vi "AWG_init.vi"(1 "Initialize?":u64, 2 "Inst_param":T1) -> (0 "error out":errorcluster)   [LabVIEW 2013]
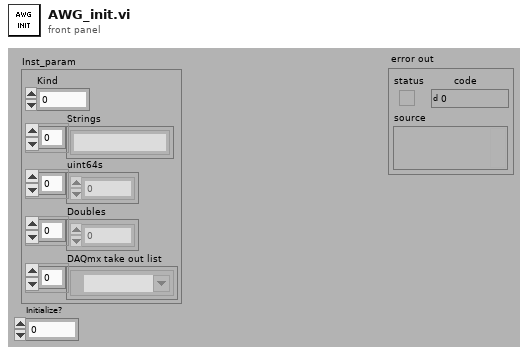
[diagram p1: front panel]
types:
  T1 = cluster{"Kind":u16, "Strings":string[], "uint64s":u64[], "Doubles":dbl[], "DAQmx take out list":refnum<k21>[]}
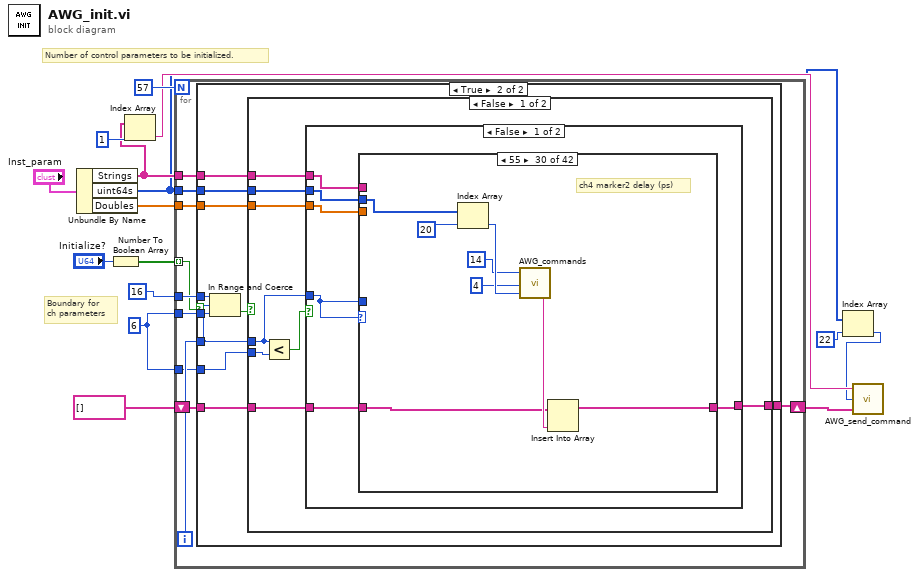
[diagram p0: block diagram]
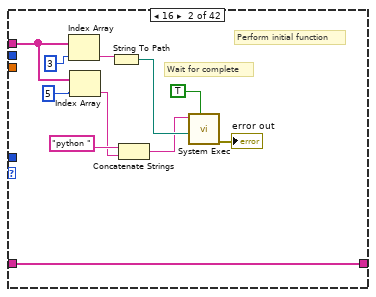
[diagram p4: hidden frame]
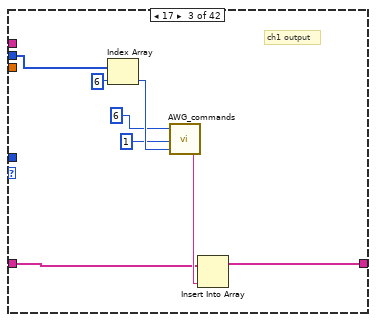
[diagram p5: hidden frame]
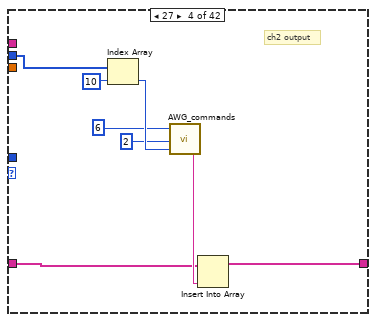
[diagram p6: hidden frame]
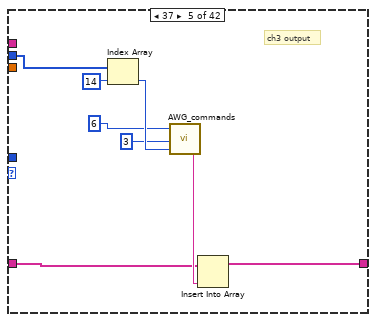
[diagram p7: hidden frame]
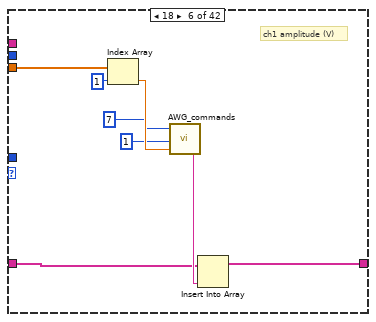
[diagram p8: hidden frame]
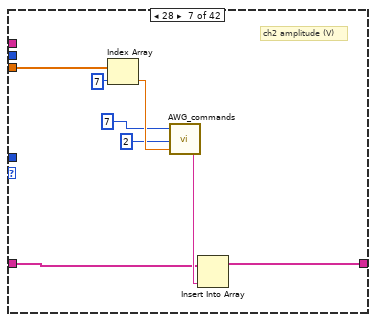
[diagram p9: hidden frame]
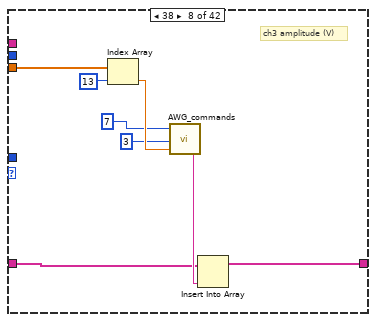
[diagram p10: hidden frame]
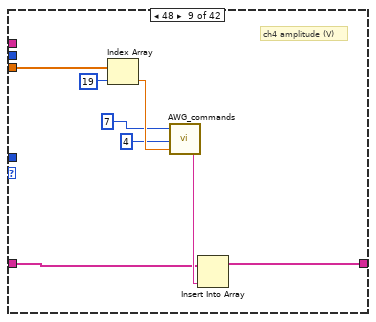
[diagram p11: hidden frame]
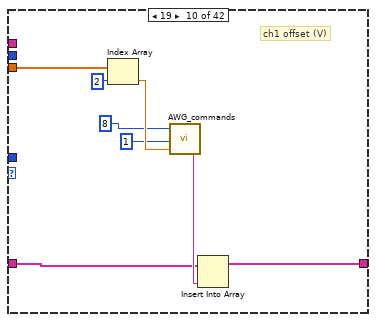
[diagram p12: hidden frame]
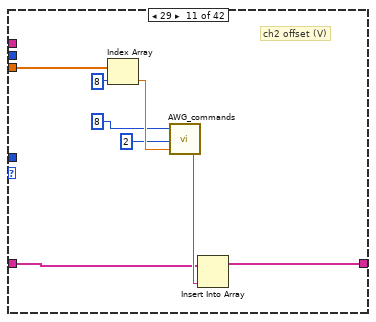
[diagram p13: hidden frame]
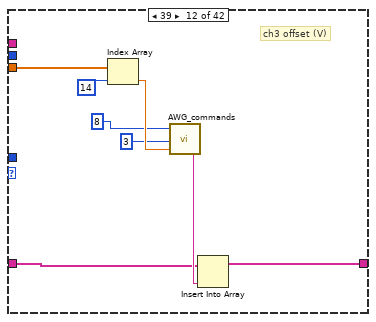
[diagram p14: hidden frame]
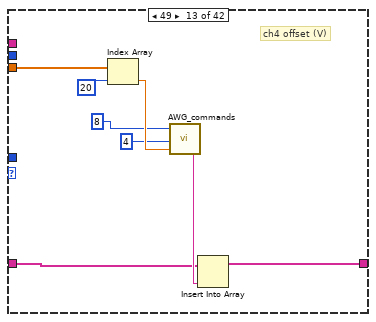
[diagram p15: hidden frame]
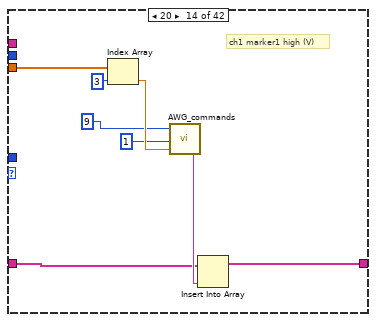
[diagram p16: hidden frame]
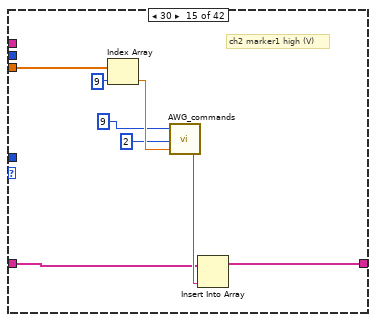
[diagram p17: hidden frame]
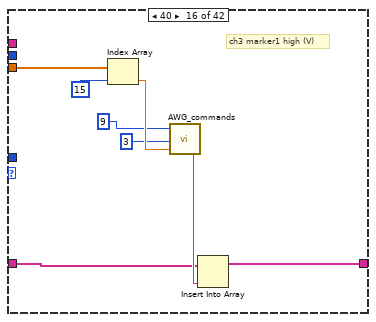
[diagram p18: hidden frame]
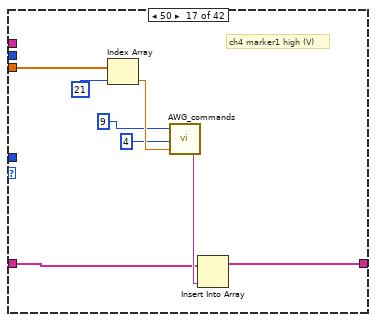
[diagram p19: hidden frame]
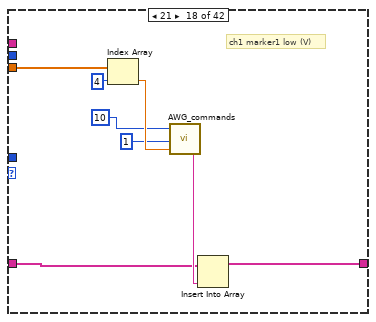
[diagram p20: hidden frame]
diagram:
  w9 = 6
  # "Boundary for\nch parameters"
  # "Number of control parameters to be initialized."
  n1 = Unbundle By Name("Inst_param") -> ("Strings"=w5:string[], "uint64s"=w2:u64[], "Doubles"=w11:dbl[])
  n2 = Number To Boolean Array(number="Initialize?") -> (Boolean array=w13:bool[])
  n3 = Index Array(array=w5, index=1) -> (element=w4:string)
  n4 = for {
    N: 57 -> [_]
    tunnel: w13 -> [w21] mode=indexing
    tunnel: w5 -> [w20]
    tunnel: w2 -> [w19]
    tunnel: w11 -> [w18]
    tunnel: w9 -> [w25]
    tunnel: 16 -> [w24]
    tunnel: w9 -> [w22]
    shift-right: [w16] -> w7
    shift-left: string[] [] -> [w17]
    i -> [w23]
    n5 = case shown="True" w21 {
      tunnel: w25 -> [_ w35]
      tunnel: w24 -> [_ w34]
      tunnel: w23 -> [_ w33]
      tunnel: w22 -> [_ w32]
      tunnel: w20 -> [_ w31]
      tunnel: w19 -> [_ w30]
      tunnel: w18 -> [_ w29]
      tunnel: w17 -> [w26 w28]
      tunnel: [w26 w27] -> w16
      frame False {
      }
      frame True {
        n6 = In Range and Coerce(upper limit=w34, x=w33, lower limit=w35) -> (In Range?=w36:bool)  [unwired: 1 out]
        n7 = case shown="False" w36 {
          tunnel: w33 -> [w42 w415]
          tunnel: w32 -> [w44 _]
          tunnel: w31 -> [w41 _]
          tunnel: w30 -> [w40 w414]
          tunnel: w29 -> [w39 w412]
          tunnel: w28 -> [w38 w413]
          tunnel: [w37 w411] -> w27
          frame False {
            n8 = Less?(x=w42, y=w44) -> (x < y?=w43:bool)
            n9 = case shown="False" w43 {
              tunnel: w42 -> [w46 w385]
              tunnel: w41 -> [w50 w388]
              tunnel: w40 -> [w45 w387]
              tunnel: w39 -> [w47 w386]
              tunnel: w38 -> [w49 w384]
              tunnel: [w48 w383] -> w37
              frame False {
                n10 = case shown="55" w46 {
                  tunnel: w50 -> [_ w62 _ _ _ _ _ _ _ _ _ _ _ _ _ _ _ _ _ _ _ _ _ _ _ _ _ _ _ _ _ _ _ _ _ _ _ _ _ _ _ _]
                  tunnel: [w51 w54 w66 w74 w82 w90 w98 w106 w114 w122 w130 w138 w146 w154 w162 w170 w178 w186 w194 w202 w210 w218 w226 w234 w242 w250 w258 w266 w274 w282 w290 w298 w306 w314 w322 w330 w338 w346 w354 w362 w370 w378] -> w48
                  tunnel: w49 -> [w51 w54 w67 w75 w83 w91 w99 w107 w115 w123 w131 w139 w147 w155 w163 w171 w179 w187 w195 w203 w211 w219 w227 w235 w243 w251 w259 w267 w275 w283 w291 w299 w307 w315 w323 w331 w339 w347 w355 w363 w371 w379]
                  tunnel: w47 -> [_ _ _ _ _ w88 w96 w104 w112 w120 w128 w136 w144 w152 w160 w168 w176 w184 w192 w200 w208 _ _ _ _ _ _ _ _ _ _ _ _ _ w320 w328 w336 w344 w352 w360 w368 w376]
                  tunnel: w46 -> [_ _ _ _ _ _ _ _ _ _ _ _ _ _ _ _ _ _ _ _ _ _ _ _ _ _ _ _ _ _ _ _ _ _ _ _ _ _ _ _ _ _]
                  tunnel: w45 -> [_ _ w65 w73 w81 _ _ _ _ _ _ _ _ _ _ _ _ _ _ _ _ w216 w224 w232 w241 w248 w256 w264 w272 w280 w288 w296 w304 w312 _ _ _ _ _ _ _ _]
                  frame 1000, Default {
                  }
                  frame 16 {
                    # "Wait for complete"
                    # "Perform initial function"
                    n11 = Index Array(array=w62, index=3) -> (element=w59:string)
                    n12 = Index Array(array=w62, index=5) -> (element=w56:string)
                    n13 = String To Path(string=w59) -> (path=w58:path)
                    n14 = Concatenate Strings("python ", w56) -> (w55:string)
                    n15 = call <vilib>:"System Exec.vi"("wait until completion? (T)"=TRUE, "working directory"=w58, "command line"=w55) -> ("error out"=→"error out":errorcluster)  [unwired: 5 in, 3 out]
                  }
                  frame 17 {
                    # "ch1 output"
                    n16 = Index Array(array=w65, index=6) -> (element=w70:u64)
                    n17 = call "AWG_commands.vi"("Value"=w70, "Channel"=1, "Commands"=6) -> ("Comannd string"=w69:string)
                    n18 = Insert Into Array(array=w67, new element=w69) -> (w66:string[])  [unwired: 1 in]
                  }
                  frame 27 {
                    # "ch2 output"
                    n19 = Index Array(array=w73, index=10) -> (element=w78:u64)
                    n20 = call "AWG_commands.vi"("Value"=w78, "Channel"=2, "Commands"=6) -> ("Comannd string"=w77:string)
                    n21 = Insert Into Array(array=w75, new element=w77) -> (w74:string[])  [unwired: 1 in]
                  }
                  frame 37 {
                    # "ch3 output"
                    n22 = Index Array(array=w81, index=14) -> (element=w86:u64)
                    n23 = call "AWG_commands.vi"("Value"=w86, "Channel"=3, "Commands"=6) -> ("Comannd string"=w85:string)
                    n24 = Insert Into Array(array=w83, new element=w85) -> (w82:string[])  [unwired: 1 in]
                  }
                  frame 18 {
                    # "ch1 amplitude (V)"
                    n25 = Index Array(array=w88, index=1) -> (element=w94:dbl)
                    n26 = call "AWG_commands.vi"("Value"=w94, "Channel"=1, "Commands"=7) -> ("Comannd string"=w93:string)
                    n27 = Insert Into Array(array=w91, new element=w93) -> (w90:string[])  [unwired: 1 in]
                  }
                  frame 28 {
                    # "ch2 amplitude (V)"
                    n28 = Index Array(array=w96, index=7) -> (element=w102:dbl)
                    n29 = call "AWG_commands.vi"("Value"=w102, "Channel"=2, "Commands"=7) -> ("Comannd string"=w101:string)
                    n30 = Insert Into Array(array=w99, new element=w101) -> (w98:string[])  [unwired: 1 in]
                  }
                  frame 38 {
                    # "ch3 amplitude (V)"
                    n31 = Index Array(array=w104, index=13) -> (element=w110:dbl)
                    n32 = call "AWG_commands.vi"("Value"=w110, "Channel"=3, "Commands"=7) -> ("Comannd string"=w109:string)
                    n33 = Insert Into Array(array=w107, new element=w109) -> (w106:string[])  [unwired: 1 in]
                  }
                  frame 48 {
                    # "ch4 amplitude (V)"
                    n34 = Index Array(array=w112, index=19) -> (element=w118:dbl)
                    n35 = call "AWG_commands.vi"("Value"=w118, "Channel"=4, "Commands"=7) -> ("Comannd string"=w117:string)
                    n36 = Insert Into Array(array=w115, new element=w117) -> (w114:string[])  [unwired: 1 in]
                  }
                  frame 19 {
                    # "ch1 offset (V)"
                    n37 = Index Array(array=w120, index=2) -> (element=w126:dbl)
                    n38 = call "AWG_commands.vi"("Value"=w126, "Channel"=1, "Commands"=8) -> ("Comannd string"=w125:string)
                    n39 = Insert Into Array(array=w123, new element=w125) -> (w122:string[])  [unwired: 1 in]
                  }
                  frame 29 {
                    # "ch2 offset (V)"
                    n40 = Index Array(array=w128, index=8) -> (element=w134:dbl)
                    n41 = call "AWG_commands.vi"("Value"=w134, "Channel"=2, "Commands"=8) -> ("Comannd string"=w133:string)
                    n42 = Insert Into Array(array=w131, new element=w133) -> (w130:string[])  [unwired: 1 in]
                  }
                  frame 39 {
                    # "ch3 offset (V)"
                    n43 = Index Array(array=w136, index=14) -> (element=w142:dbl)
                    n44 = call "AWG_commands.vi"("Value"=w142, "Channel"=3, "Commands"=8) -> ("Comannd string"=w141:string)
                    n45 = Insert Into Array(array=w139, new element=w141) -> (w138:string[])  [unwired: 1 in]
                  }
                  frame 49 {
                    # "ch4 offset (V)"
                    n46 = Index Array(array=w144, index=20) -> (element=w150:dbl)
                    n47 = call "AWG_commands.vi"("Value"=w150, "Channel"=4, "Commands"=8) -> ("Comannd string"=w149:string)
                    n48 = Insert Into Array(array=w147, new element=w149) -> (w146:string[])  [unwired: 1 in]
                  }
                  frame 20 {
                    # "ch1 marker1 high (V)"
                    n49 = Index Array(array=w152, index=3) -> (element=w158:dbl)
                    n50 = call "AWG_commands.vi"("Value"=w158, "Channel"=1, "Commands"=9) -> ("Comannd string"=w157:string)
                    n51 = Insert Into Array(array=w155, new element=w157) -> (w154:string[])  [unwired: 1 in]
                  }
                  frame 30 {
                    # "ch2 marker1 high (V)"
                    n52 = Index Array(array=w160, index=9) -> (element=w166:dbl)
                    n53 = call "AWG_commands.vi"("Value"=w166, "Channel"=2, "Commands"=9) -> ("Comannd string"=w165:string)
                    n54 = Insert Into Array(array=w163, new element=w165) -> (w162:string[])  [unwired: 1 in]
                  }
                  frame 40 {
                    # "ch3 marker1 high (V)"
                    n55 = Index Array(array=w168, index=15) -> (element=w174:dbl)
                    n56 = call "AWG_commands.vi"("Value"=w174, "Channel"=3, "Commands"=9) -> ("Comannd string"=w173:string)
                    n57 = Insert Into Array(array=w171, new element=w173) -> (w170:string[])  [unwired: 1 in]
                  }
                  frame 50 {
                    # "ch4 marker1 high (V)"
                    n58 = Index Array(array=w176, index=21) -> (element=w182:dbl)
                    n59 = call "AWG_commands.vi"("Value"=w182, "Channel"=4, "Commands"=9) -> ("Comannd string"=w181:string)
                    n60 = Insert Into Array(array=w179, new element=w181) -> (w178:string[])  [unwired: 1 in]
                  }
                  frame 21 {
                    # "ch1 marker1 low (V)"
                    n61 = Index Array(array=w184, index=4) -> (element=w190:dbl)
                    n62 = call "AWG_commands.vi"("Value"=w190, "Channel"=1, "Commands"=10) -> ("Comannd string"=w189:string)
                    n63 = Insert Into Array(array=w187, new element=w189) -> (w186:string[])  [unwired: 1 in]
                  }
                  frame 31 {
                    # "ch2 marker1 low (V)"
                    n64 = Index Array(array=w192, index=10) -> (element=w198:dbl)
                    n65 = call "AWG_commands.vi"("Value"=w198, "Channel"=2, "Commands"=10) -> ("Comannd string"=w197:string)
                    n66 = Insert Into Array(array=w195, new element=w197) -> (w194:string[])  [unwired: 1 in]
                  }
                  frame 41 {
                    # "ch3 marker1 low (V)"
                    n67 = Index Array(array=w200, index=16) -> (element=w206:dbl)
                    n68 = call "AWG_commands.vi"("Value"=w206, "Channel"=3, "Commands"=10) -> ("Comannd string"=w205:string)
                    n69 = Insert Into Array(array=w203, new element=w205) -> (w202:string[])  [unwired: 1 in]
                  }
                  frame 51 {
                    # "ch4 marker1 low (V)"
                    n70 = Index Array(array=w208, index=22) -> (element=w214:dbl)
                    n71 = call "AWG_commands.vi"("Value"=w214, "Channel"=4, "Commands"=10) -> ("Comannd string"=w213:string)
                    n72 = Insert Into Array(array=w211, new element=w213) -> (w210:string[])  [unwired: 1 in]
                  }
                  frame 22 {
                    # "ch1 marker1 delay (ps)"
                    n73 = Index Array(array=w216, index=7) -> (element=w222:u64)
                    n74 = call "AWG_commands.vi"("Value"=w222, "Channel"=1, "Commands"=11) -> ("Comannd string"=w221:string)
                    n75 = Insert Into Array(array=w219, new element=w221) -> (w218:string[])  [unwired: 1 in]
                  }
                  frame 32 {
                    # "ch2 marker1 delay (ps)"
                    n76 = Index Array(array=w224, index=11) -> (element=w230:u64)
                    n77 = call "AWG_commands.vi"("Value"=w230, "Channel"=2, "Commands"=11) -> ("Comannd string"=w229:string)
                    n78 = Insert Into Array(array=w227, new element=w229) -> (w226:string[])  [unwired: 1 in]
                  }
                  frame 42 {
                    # "ch3 marker1 delay (ps)"
                    n79 = Index Array(array=w232, index=15) -> (element=w238:u64)
                    n80 = call "AWG_commands.vi"("Value"=w238, "Channel"=3, "Commands"=11) -> ("Comannd string"=w237:string)
                    n81 = Insert Into Array(array=w235, new element=w237) -> (w234:string[])  [unwired: 1 in]
                  }
                  frame 47 {
                    # "ch4 output"
                    n82 = Index Array(array=w241, index=18) -> (element=w246:u64)
                    n83 = call "AWG_commands.vi"("Value"=w246, "Channel"=4, "Commands"=6) -> ("Comannd string"=w245:string)
                    n84 = Insert Into Array(array=w243, new element=w245) -> (w242:string[])  [unwired: 1 in]
                  }
                  frame 52 {
                    # "ch4 marker1 delay (ps)"
                    n85 = Index Array(array=w248, index=19) -> (element=w254:u64)
                    n86 = call "AWG_commands.vi"("Value"=w254, "Channel"=4, "Commands"=11) -> ("Comannd string"=w253:string)
                    n87 = Insert Into Array(array=w251, new element=w253) -> (w250:string[])  [unwired: 1 in]
                  }
                  frame 25 {
                    # "ch1 marker2 delay (ps)"
                    n88 = Index Array(array=w256, index=8) -> (element=w262:u64)
                    n89 = call "AWG_commands.vi"("Value"=w262, "Channel"=1, "Commands"=14) -> ("Comannd string"=w261:string)
                    n90 = Insert Into Array(array=w259, new element=w261) -> (w258:string[])  [unwired: 1 in]
                  }
                  frame 35 {
                    # "ch2 marker2 delay (ps)"
                    n91 = Index Array(array=w264, index=12) -> (element=w270:u64)
                    n92 = call "AWG_commands.vi"("Value"=w270, "Channel"=2, "Commands"=14) -> ("Comannd string"=w269:string)
                    n93 = Insert Into Array(array=w267, new element=w269) -> (w266:string[])  [unwired: 1 in]
                  }
                  frame 45 {
                    # "ch3 marker2 delay (ps)"
                    n94 = Index Array(array=w272, index=16) -> (element=w278:u64)
                    n95 = call "AWG_commands.vi"("Value"=w278, "Channel"=3, "Commands"=14) -> ("Comannd string"=w277:string)
                    n96 = Insert Into Array(array=w275, new element=w277) -> (w274:string[])  [unwired: 1 in]
                  }
                  frame 55 {
                    # "ch4 marker2 delay (ps)"
                    n97 = Index Array(array=w280, index=20) -> (element=w286:u64)
                    n98 = call "AWG_commands.vi"("Value"=w286, "Channel"=4, "Commands"=14) -> ("Comannd string"=w285:string)
                    n99 = Insert Into Array(array=w283, new element=w285) -> (w282:string[])  [unwired: 1 in]
                  }
                  frame 26 {
                    # "ch1 skew (ps)"
                    n100 = Index Array(array=w288, index=9) -> (element=w294:u64)
                    n101 = call "AWG_commands.vi"("Value"=w294, "Channel"=1, "Commands"=15) -> ("Comannd string"=w293:string)
                    n102 = Insert Into Array(array=w291, new element=w293) -> (w290:string[])  [unwired: 1 in]
                  }
                  frame 36 {
                    # "ch2 skew (ps)"
                    n103 = Index Array(array=w296, index=13) -> (element=w302:u64)
                    n104 = call "AWG_commands.vi"("Value"=w302, "Channel"=2, "Commands"=15) -> ("Comannd string"=w301:string)
                    n105 = Insert Into Array(array=w299, new element=w301) -> (w298:string[])  [unwired: 1 in]
                  }
                  frame 46 {
                    # "ch3 skew (ps)"
                    n106 = Index Array(array=w304, index=17) -> (element=w310:u64)
                    n107 = call "AWG_commands.vi"("Value"=w310, "Channel"=3, "Commands"=15) -> ("Comannd string"=w309:string)
                    n108 = Insert Into Array(array=w307, new element=w309) -> (w306:string[])  [unwired: 1 in]
                  }
                  frame 56 {
                    # "ch4 skew (ps)"
                    n109 = Index Array(array=w312, index=21) -> (element=w318:u64)
                    n110 = call "AWG_commands.vi"("Value"=w318, "Channel"=4, "Commands"=15) -> ("Comannd string"=w317:string)
                    n111 = Insert Into Array(array=w315, new element=w317) -> (w314:string[])  [unwired: 1 in]
                  }
                  frame 23 {
                    # "ch1 marker2 high (V)"
                    n112 = Index Array(array=w320, index=5) -> (element=w326:dbl)
                    n113 = call "AWG_commands.vi"("Value"=w326, "Channel"=1, "Commands"=12) -> ("Comannd string"=w325:string)
                    n114 = Insert Into Array(array=w323, new element=w325) -> (w322:string[])  [unwired: 1 in]
                  }
                  frame 33 {
                    # "ch2 marker2 high (V)"
                    n115 = Index Array(array=w328, index=11) -> (element=w334:dbl)
                    n116 = call "AWG_commands.vi"("Value"=w334, "Channel"=2, "Commands"=12) -> ("Comannd string"=w333:string)
                    n117 = Insert Into Array(array=w331, new element=w333) -> (w330:string[])  [unwired: 1 in]
                  }
                  frame 43 {
                    # "ch3 marker2 high (V)"
                    n118 = Index Array(array=w336, index=17) -> (element=w342:dbl)
                    n119 = call "AWG_commands.vi"("Value"=w342, "Channel"=3, "Commands"=12) -> ("Comannd string"=w341:string)
                    n120 = Insert Into Array(array=w339, new element=w341) -> (w338:string[])  [unwired: 1 in]
                  }
                  frame 53 {
                    # "ch4 marker2 high (V)"
                    n121 = Index Array(array=w344, index=23) -> (element=w350:dbl)
                    n122 = call "AWG_commands.vi"("Value"=w350, "Channel"=4, "Commands"=12) -> ("Comannd string"=w349:string)
                    n123 = Insert Into Array(array=w347, new element=w349) -> (w346:string[])  [unwired: 1 in]
                  }
                  frame 24 {
                    # "ch1 marker2 low (V)"
                    n124 = Index Array(array=w352, index=6) -> (element=w358:dbl)
                    n125 = call "AWG_commands.vi"("Value"=w358, "Channel"=1, "Commands"=13) -> ("Comannd string"=w357:string)
                    n126 = Insert Into Array(array=w355, new element=w357) -> (w354:string[])  [unwired: 1 in]
                  }
                  frame 34 {
                    # "ch2 marker2 low (V)"
                    n127 = Index Array(array=w360, index=12) -> (element=w366:dbl)
                    n128 = call "AWG_commands.vi"("Value"=w366, "Channel"=2, "Commands"=13) -> ("Comannd string"=w365:string)
                    n129 = Insert Into Array(array=w363, new element=w365) -> (w362:string[])  [unwired: 1 in]
                  }
                  frame 44 {
                    # "ch3 marker2 low (V)"
                    n130 = Index Array(array=w368, index=18) -> (element=w374:dbl)
                    n131 = call "AWG_commands.vi"("Value"=w374, "Channel"=3, "Commands"=13) -> ("Comannd string"=w373:string)
                    n132 = Insert Into Array(array=w371, new element=w373) -> (w370:string[])  [unwired: 1 in]
                  }
                  frame 54 {
                    # "ch4 marker2 low (V)"
                    n133 = Index Array(array=w376, index=24) -> (element=w382:dbl)
                    n134 = call "AWG_commands.vi"("Value"=w382, "Channel"=4, "Commands"=13) -> ("Comannd string"=w381:string)
                    n135 = Insert Into Array(array=w379, new element=w381) -> (w378:string[])  [unwired: 1 in]
                  }
                }
              }
              frame True {
                n136 = case shown="3" w385 {
                  tunnel: w388 -> [_ _ _ _]
                  tunnel: w387 -> [_ w391 w398 _]
                  tunnel: w386 -> [_ _ _ w404]
                  tunnel: w385 -> [_ w396 w403 w410]
                  tunnel: w384 -> [w389 w394 w401 w408]
                  tunnel: [w389 w393 w400 w407] -> w383
                  frame 1000, Default {
                  }
                  frame 0 {
                    # "Run ??"
                    n137 = Index Array(array=w391, index=2) -> (element=w390:u64)
                    n138 = call "AWG_commands.vi"("Value"=w390, "Commands"=w396) -> ("Comannd string"=w392:string)  [unwired: 1 in]
                    n139 = Insert Into Array(array=w394, new element=w392) -> (w393:string[])  [unwired: 1 in]
                  }
                  frame 2 {
                    # "Run mode"
                    n140 = Index Array(array=w398, index=3) -> (element=w397:u64)
                    n141 = call "AWG_commands.vi"("Value"=w397, "Commands"=w403) -> ("Comannd string"=w399:string)  [unwired: 1 in]
                    n142 = Insert Into Array(array=w401, new element=w399) -> (w400:string[])  [unwired: 1 in]
                  }
                  frame 3 {
                    # "Sampling frequency"
                    n143 = Index Array(array=w404, index=0) -> (element=w405:dbl)
                    n144 = call "AWG_commands.vi"("Value"=w405, "Commands"=w410) -> ("Comannd string"=w406:string)  [unwired: 1 in]
                    n145 = Insert Into Array(array=w408, new element=w406) -> (w407:string[])  [unwired: 1 in]
                  }
                }
              }
            }
          }
          frame True {
            # "No of channels to be used"
            n146 = Index Array(array=w414, index=0) -> (element=w416:u64)
            n147 = for {
              N: w416 -> [_]
              tunnel: w415 -> [w422]
              tunnel: w414 -> [w421]
              tunnel: w412 -> [w419]
              shift-right: [w418] -> w411
              shift-left: w413 -> [w420]
              i -> [w423]
              n148 = case shown="8" w422 {
                tunnel: w423 -> [_ w434 w446 w458 w470 w482 w494 w506 w518 w530 w542]
                tunnel: w422 -> [_ w431 w443 w455 w467 w479 w491 w503 w515 w527 w539]
                tunnel: w421 -> [_ w429 _ _ _ _ w485 _ _ w521 w533]
                tunnel: w420 -> [w424 w427 w440 w452 w464 w476 w488 w500 w512 w524 w536]
                tunnel: [w424 w426 w439 w451 w463 w475 w487 w499 w511 w523 w535] -> w418
                tunnel: w419 -> [_ _ w437 w449 w461 w473 _ w497 w509 _ _]
                frame 1000, Default {
                }
                frame 6 {
                  # "Ch output on?"
                  n149 = Increment(x=w434) -> (x+1=w436:i32)
                  n150 = Multiply(x=4, y=w434) -> (x*y=w435:i32)
                  n151 = Add(x=6, y=w435) -> (x+y=w430:i32)
                  n152 = Index Array(array=w429, index=w430) -> (element=w428:u64)
                  n153 = call "AWG_commands.vi"("Value"=w428, "Channel"=w436, "Commands"=w431) -> ("Comannd string"=w425:string)
                  n154 = Insert Into Array(array=w427, new element=w425) -> (w426:string[])  [unwired: 1 in]
                }
                frame 7 {
                  # "ch amplitude (V)"
                  n155 = Increment(x=w446) -> (x+1=w448:i32)
                  n156 = Multiply(x=6, y=w446) -> (x*y=w447:i32)
                  n157 = Add(x=1, y=w447) -> (x+y=w442:i32)
                  n158 = Index Array(array=w437, index=w442) -> (element=w441:dbl)
                  n159 = call "AWG_commands.vi"("Value"=w441, "Channel"=w448, "Commands"=w443) -> ("Comannd string"=w438:string)
                  n160 = Insert Into Array(array=w440, new element=w438) -> (w439:string[])  [unwired: 1 in]
                }
                frame 8 {
                  # "ch offset voltage (V)"
                  n161 = Increment(x=w458) -> (x+1=w460:i32)
                  n162 = Multiply(x=6, y=w458) -> (x*y=w459:i32)
                  n163 = Add(x=2, y=w459) -> (x+y=w454:i32)
                  n164 = Index Array(array=w449, index=w454) -> (element=w453:dbl)
                  n165 = call "AWG_commands.vi"("Value"=w453, "Channel"=w460, "Commands"=w455) -> ("Comannd string"=w450:string)
                  n166 = Insert Into Array(array=w452, new element=w450) -> (w451:string[])  [unwired: 1 in]
                }
                frame 9 {
                  # "ch marker1 high (V)"
                  n167 = Increment(x=w470) -> (x+1=w472:i32)
                  n168 = Multiply(x=6, y=w470) -> (x*y=w471:i32)
                  n169 = Add(x=3, y=w471) -> (x+y=w466:i32)
                  n170 = Index Array(array=w461, index=w466) -> (element=w465:dbl)
                  n171 = call "AWG_commands.vi"("Value"=w465, "Channel"=w472, "Commands"=w467) -> ("Comannd string"=w462:string)
                  n172 = Insert Into Array(array=w464, new element=w462) -> (w463:string[])  [unwired: 1 in]
                }
                frame 10 {
                  # "ch marker1 low (V)"
                  n173 = Increment(x=w482) -> (x+1=w484:i32)
                  n174 = Multiply(x=6, y=w482) -> (x*y=w483:i32)
                  n175 = Add(x=4, y=w483) -> (x+y=w478:i32)
                  n176 = Index Array(array=w473, index=w478) -> (element=w477:dbl)
                  n177 = call "AWG_commands.vi"("Value"=w477, "Channel"=w484, "Commands"=w479) -> ("Comannd string"=w474:string)
                  n178 = Insert Into Array(array=w476, new element=w474) -> (w475:string[])  [unwired: 1 in]
                }
                frame 11 {
                  # "ch marker1 delay (ps)"
                  n179 = Increment(x=w494) -> (x+1=w496:i32)
                  n180 = Multiply(x=4, y=w494) -> (x*y=w495:i32)
                  n181 = Add(x=7, y=w495) -> (x+y=w490:i32)
                  n182 = Index Array(array=w485, index=w490) -> (element=w489:u64)
                  n183 = call "AWG_commands.vi"("Value"=w489, "Channel"=w496, "Commands"=w491) -> ("Comannd string"=w486:string)
                  n184 = Insert Into Array(array=w488, new element=w486) -> (w487:string[])  [unwired: 1 in]
                }
                frame 12 {
                  # "ch marker2 high (V)"
                  n185 = Increment(x=w506) -> (x+1=w508:i32)
                  n186 = Multiply(x=6, y=w506) -> (x*y=w507:i32)
                  n187 = Add(x=5, y=w507) -> (x+y=w502:i32)
                  n188 = Index Array(array=w497, index=w502) -> (element=w501:dbl)
                  n189 = call "AWG_commands.vi"("Value"=w501, "Channel"=w508, "Commands"=w503) -> ("Comannd string"=w498:string)
                  n190 = Insert Into Array(array=w500, new element=w498) -> (w499:string[])  [unwired: 1 in]
                }
                frame 13 {
                  # "ch marker2 low (V)"
                  n191 = Increment(x=w518) -> (x+1=w520:i32)
                  n192 = Multiply(x=6, y=w518) -> (x*y=w519:i32)
                  n193 = Add(x=6, y=w519) -> (x+y=w514:i32)
                  n194 = Index Array(array=w509, index=w514) -> (element=w513:dbl)
                  n195 = call "AWG_commands.vi"("Value"=w513, "Channel"=w520, "Commands"=w515) -> ("Comannd string"=w510:string)
                  n196 = Insert Into Array(array=w512, new element=w510) -> (w511:string[])  [unwired: 1 in]
                }
                frame 14 {
                  # "ch marker2 delay (ps)"
                  n197 = Increment(x=w530) -> (x+1=w532:i32)
                  n198 = Multiply(x=4, y=w530) -> (x*y=w531:i32)
                  n199 = Add(x=8, y=w531) -> (x+y=w526:i32)
                  n200 = Index Array(array=w521, index=w526) -> (element=w525:u64)
                  n201 = call "AWG_commands.vi"("Value"=w525, "Channel"=w532, "Commands"=w527) -> ("Comannd string"=w522:string)
                  n202 = Insert Into Array(array=w524, new element=w522) -> (w523:string[])  [unwired: 1 in]
                }
                frame 15 {
                  # "ch skew (ps)"
                  n203 = Increment(x=w542) -> (x+1=w544:i32)
                  n204 = Multiply(x=4, y=w542) -> (x*y=w543:i32)
                  n205 = Add(x=9, y=w543) -> (x+y=w538:i32)
                  n206 = Index Array(array=w533, index=w538) -> (element=w537:u64)
                  n207 = call "AWG_commands.vi"("Value"=w537, "Channel"=w544, "Commands"=w539) -> ("Comannd string"=w534:string)
                  n208 = Insert Into Array(array=w536, new element=w534) -> (w535:string[])  [unwired: 1 in]
                }
              }
            }
          }
        }
      }
    }
  }
  n209 = Index Array(array=w2, index=22) -> (element=w1:u64)
  n210 = call "AWG_send_command.vi"("CMD list"=w7, "Port number"=w1, "IP Address"=w4) -> ()  [unwired: 1 in]
